vi "Table Sav for NG.vi"(8 "error in (no error)":errorcluster, 11 "SN":string="07") -> (0 "error out":errorcluster, 3 "未找到條碼":bool)   [LabVIEW 2019]
uses:
  Ctrl/Table Save.ctl
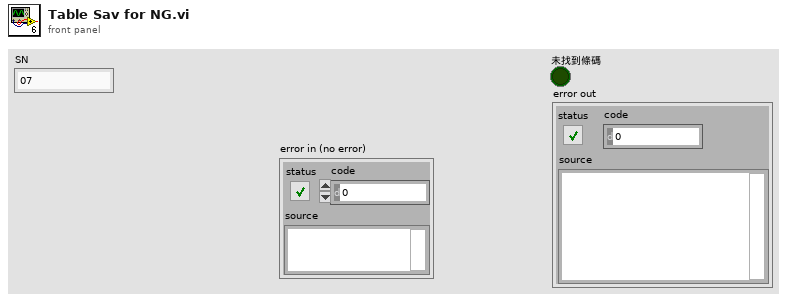
[diagram p1: front panel]
types:
  T1 = typedef "Table Save.ctl" = enum16{"initial", "Add", "Write", "Replace", "Delete", "REad", "RedTable", "Load"}
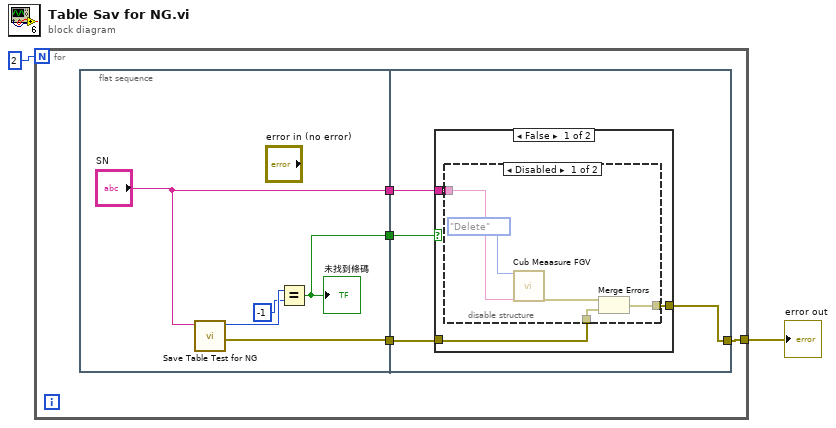
[diagram p0: block diagram]
diagram:
  n1 = for {
    N: 2 -> [_]
    tunnel: [w4] -> w2
    n2 = flat-sequence {
      tunnel: [w9] -> w6
      tunnel: ["SN"] -> w5
      tunnel: [w7] -> w3
      tunnel: [w13] -> w4
      tunnel: w6 -> [w14]
      tunnel: w5 -> [w15]
      tunnel: w3 -> [w12]
      frame #0 {
        n3 = call "Save Table Test for NG.vi"("SN"="SN") -> ("error out"=w9:errorcluster, "條碼的Index"=w11:i32)  [unwired: 9 in]
        n4 = Equal?(x=w11, y=-1) -> (x = y?=w7:bool)
        "未找到條碼" <- w7
      }
      frame #1 {
        n5 = case shown="False" w12 {
          tunnel: w15 -> [w18 _]
          tunnel: w14 -> [w17 w25]
          tunnel: [w16 w25] -> w13
          frame False {
            n6 = disable-structure shown="Disabled" {
              disable-tunnel: w18 -> [w23 _]
              disable-tunnel: w17 -> [w20 w24]
              disable-tunnel: [w19 w24] -> w16
              frame Disabled {
                n7 = call "Cub Meaasure FGV.vi"("Action"=Table_Save."Delete", "SN"=w23) -> ("error out"=w21:errorcluster)  [unwired: 10 in, 7 out]
                n8 = Merge Errors(w21, w20) -> (w19:errorcluster)
              }
              frame Enabled {
              }
            }
          }
          frame True {
          }
        }
      }
    }
  }
  "error out" <- w2
